vi "FGV Zuordnungstabelle Vis PNS.vi"(6 "Prozessvariable Nr. N":i16, 7 "Initialisieren":bool, 8 "Wert (N)":string, 9 "Zuordnungtabelle (init)":i16[][](array[numeric]), 10 "Programm (init)":T1[](array[typedef])) -> (0 "Wert für zeichnen":string, 1 "Zeichenbefehle":T1[](array[typedef]), 3 "Stellung x":i16)   [LabVIEW 2020, in "Anlagenuebersicht.lvlib"]
doc: "Übernimmt als Funktionale Globale Variable im Zustand \"Initialisieren\" die Zuordnungstabelle und das Bewegtprogramm einer Visualisierung.\n\nFür die laufende Darstellung der Grafik wird entsprechend \"Wert (N)\", dem aktuellen Wert der Prozessvariablen Nr.N, jene Sequenz von Zeichenbefehlen (mit Parametern) bereitgestellt, die zur Darstellung der Prozessvariablen Nr. N in der aktuellen Stellung x gebraucht werden.\n\nFür Zeichenbefehle (wie zB. Ziffernanzeigen, variabler Text), die einen Zahlenwert oder String brauchen, steht der zugehörige Wert mit korrekter Anzahl von Nachkommastellen in \"Wert für zeichnen\" bereit."
uses:
  Anlagenuebersicht.lvlib
  VisParameter/VisSchritt.ctl
  VisParameter/VisSchritt-Typ.ctl
  VisBx Anzeige.lvlib
  VisParameter/VisParam-Typdef.lvlib
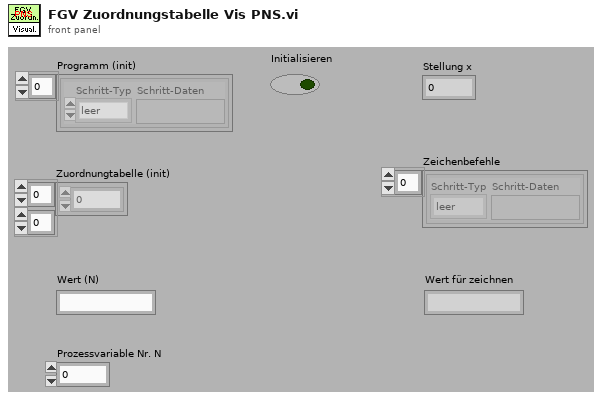
[diagram p1: front panel]
types:
  T1 = typedef "VisParam-Typdef.lvlib/VisSchritt.ctl" = cluster{"Schritt-Typ":T2, "Schritt-Daten":variant}
  T2 = typedef "VisParam-Typdef.lvlib/VisSchritt-Typ.ctl" = enum16{"leer", "Punkt", "Linie", "Linienzug", "Fixtext", "Textrechteck", "Ziffernanzeige", "Rechteck", "Rechteck rund", "Ellipse", "Bogen", "Kreis", "Pixmap"}
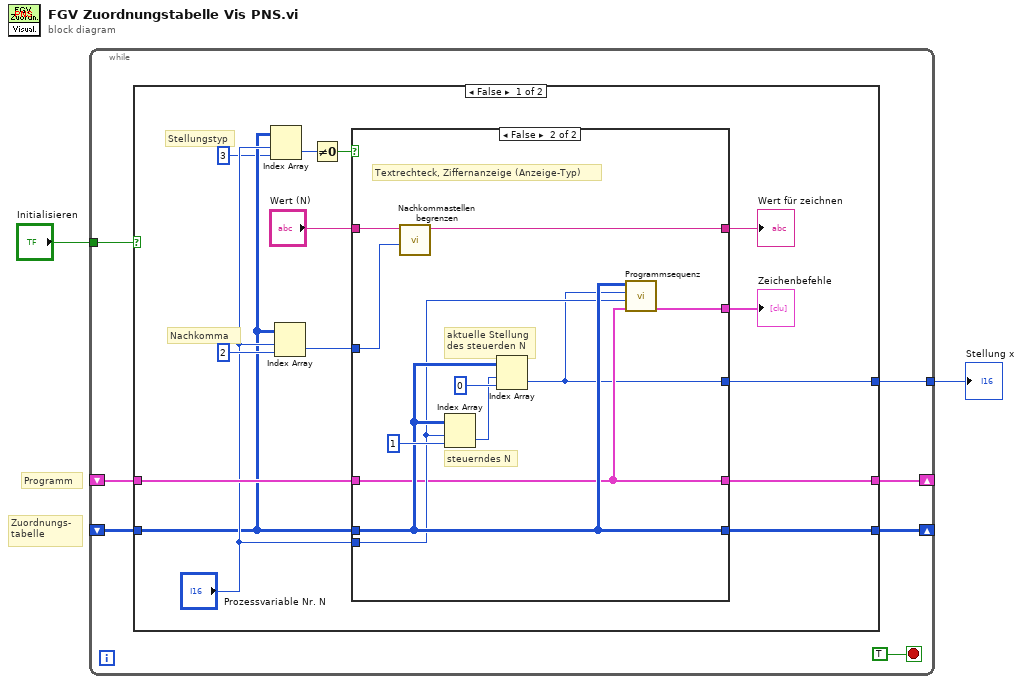
[diagram p0: block diagram]
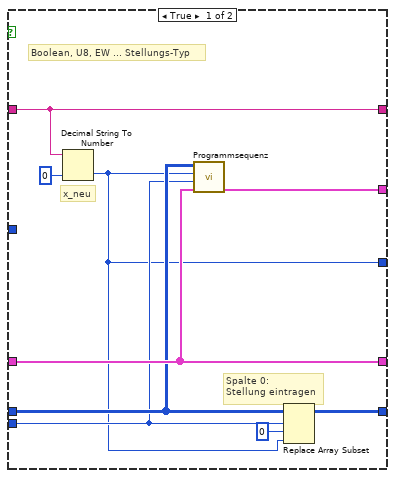
[diagram p2: hidden frame]
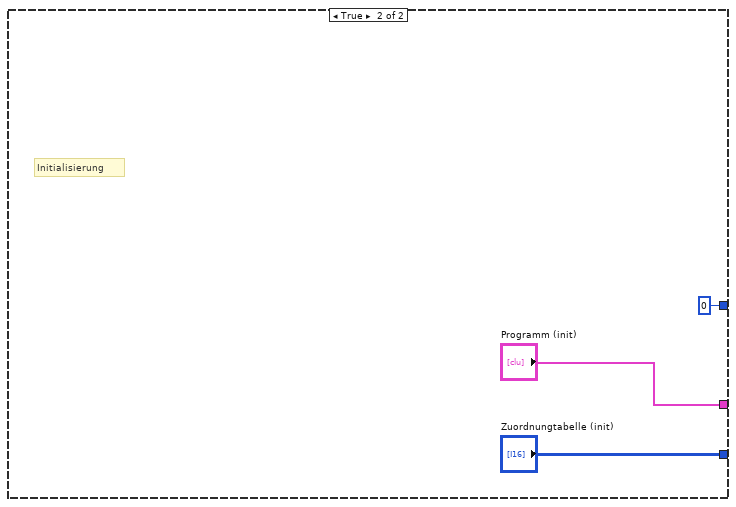
[diagram p3: hidden frame]
diagram:
  # "Programm"
  # "Zuordnungs-\ntabelle"
  n1 = while {
    shift-right: [w8] -> _
    shift-left: _ -> [w9]
    tunnel: "Initialisieren" -> [w6]
    shift-right: [w5] -> _
    shift-left: _ -> [w4]
    tunnel: [w3] -> w1
    stop <- TRUE stop-if-true
    n2 = case shown="False" w6 {
      tunnel: w9 -> [w14 _]
      tunnel: [w16 "Zuordnungtabelle (init)"] -> w8
      tunnel: [w21 "Programm (init)"] -> w5
      tunnel: w4 -> [w22 _]
      tunnel: [w10 i16 0 ("Element")] -> w3
      frame False {
        # "Stellungstyp"
        # "Nachkomma"
        n3 = Index Array(array=w14, index (row)="Prozessvariable Nr. N", index (col)=3 ("Deaktivierter Index (Spalte)")) -> (element=w11:i16)
        n4 = Index Array(array=w14, index (row)="Prozessvariable Nr. N", index (col)=2 ("Deaktivierter Index (Spalte)")) -> (element=w19:i16)
        n5 = Not Equal To 0?(x=w11) -> (x != 0?=w12:bool)
        n6 = case shown="False" w12 {
          tunnel: [w27 w38] -> w16
          tunnel: [w30 w43] -> w23
          tunnel: w22 -> [w31 w36]
          tunnel: w14 -> [w28 w38]
          tunnel: [w31 w36] -> w21
          tunnel: "Wert (N)" -> [w24 w35]
          tunnel: "Prozessvariable Nr. N" -> [w26 w37]
          tunnel: [w24 w33] -> w20
          tunnel: w19 -> [_ w39]
          tunnel: [w25 w34] -> w10
          frame True {
            # "Spalte 0: \nStellung eintragen"
            # "x_neu"
            # "Boolean, U8, EW ... Stellungs-Typ"
            n7 = Decimal String To Number(string=w24, default (0L)=i16 0 ("U16")) -> (number=w25:i16)  [unwired: 2 out]
            n8 = call "Programmsequenz.vi"("Programm"=w31, "Prozessvariable Nr. N"=w26, "Stellung x (0..9)"=w25, "Zuordnungtabelle"=w28) -> ("Sequenz"=w30:T1[])  [unwired: 7 out]
            n9 = Replace Array Subset(array=w28, new element=w25, index (row)=w26, index (col)=0 ("Deaktivierter Index (Spalte)")) -> (w27:i16[][])
          }
          frame False {
            # "aktuelle Stellung\ndes steuerden N"
            # "steuerndes N"
            # "Textrechteck, Ziffernanzeige (Anzeige-Typ)"
            n10 = call "Nachkommastellen begrenzen.vi"("Nachkommastellen"=w39, "DBL-String mit Deziamlpunkt"=w35) -> ("Anzeigestring mit Komma"=w33:string)  [unwired: 9 out]
            n11 = Index Array(array=w38, index (row)=w37, index (col)=1 ("Deaktivierter Index (Spalte)")) -> (element=w40:i16)
            n12 = Index Array(array=w38, index (row)=w40, index (col)=0 ("Deaktivierter Index (Spalte)")) -> (element=w34:i16)
            n13 = call "Programmsequenz.vi"("Programm"=w36, "Prozessvariable Nr. N"=w37, "Stellung x (0..9)"=w34, "Zuordnungtabelle"=w38) -> ("Sequenz"=w43:T1[])  [unwired: 7 out]
          }
        }
        "Zeichenbefehle" <- w23
        "Wert für zeichnen" <- w20
      }
      frame True {
        # "Initialisierung"
      }
    }
  }
  "Stellung x" <- w1
